vi "ListAttributes.vi"(6 "Inheritable Only? (F: all)":bool, 8 "error in (no error)":errorcluster, 11 "SMO in":refnum<class "SMO.lvclass">) -> (0 "error out":errorcluster, 2 "[Attributes]":refnum<class "Attribute.lvclass">[](array[class]), 3 "SMO out":refnum<class "SMO.lvclass">)   [LabVIEW 2021, in "smo.lvlib" / "SMO.lvclass"]
uses:
  SMO.lvclass
  Support/Attribute/Attribute.lvclass
  SMO.lvclass/SMO.ctl
  Support/Attribute/Attribute.lvclass/Attribute.ctl
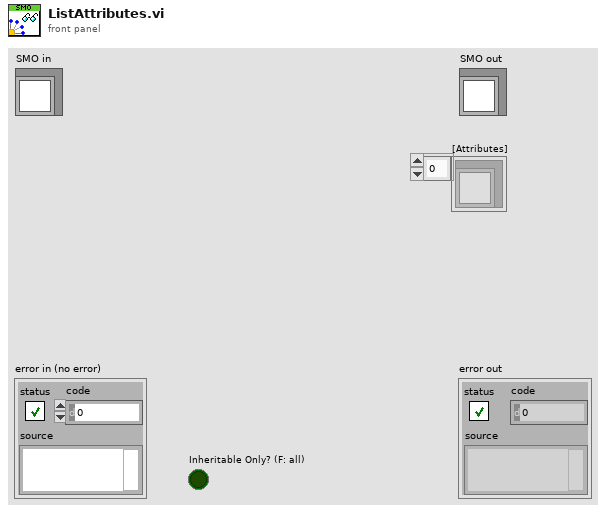
[diagram p1: front panel]
types:
  T1 = typedef "smo.lvlib/SMO.lvclass/PrivateData--Ref.ctl" = refnum<data-value>
  T2 = typedef "smo.lvlib/SMO.lvclass/PrivateData--Cluster.ctl" = cluster{"Parent Call":T3, "Registered Processes":T4[], "Sync Notifier":refnum<notifier>, "Process Error Notifier":refnum<notifier>, "Protected Events":T5, "Public Events":T6, "SMO State":T7, "[Attributes]":variant, "Launcher Close":refnum<notifier>, "Caller Watchdog":refnum<queue>, "Accessibility":T8, "NbStaticDependencies":u32}
  T3 = typedef "smo.lvlib/SMO.lvclass/Parent Call--Enum.ctl" = enum16{"Allows parent to run", "Does not request parent to run"}
  T4 = typedef "smo.lvlib/SMO.lvclass/RegisteredProcessData--Cluster.ctl" = cluster{"Name":string, "Static VI Ref":refnum<vi>, "Running":bool, "NotifierRef":u32}
  T5 = typedef "smo.lvlib/SMO.lvclass/Protected Events.ctl" = cluster{"StopProcesses":refnum<user-event>, "AbortProcesses":refnum<user-event>, "Config Changed":refnum<user-event>, "Dependency":refnum<user-event>}
  T6 = typedef "smo.lvlib/SMO.lvclass/Public Events.ctl" = cluster{"Error":refnum<user-event>, "State":refnum<user-event>, "Reserve State":refnum<user-event>}
  T7 = typedef "smo.lvlib/SMO.lvclass/SMOState --Enum.ctl" = enum16{"unknown", "Created", "Started", "Stopped"}
  T8 = typedef "smo.lvlib/SMO.lvclass/Accessibility--Cluster.ctl" = cluster{"Lock Key":string, "Reserve State":T9}
  T9 = typedef "smo.lvlib/SMO.lvclass/Reserve State--Enum.ctl" = enum16{"Unreserved", "Reserved", "Self-locked"}
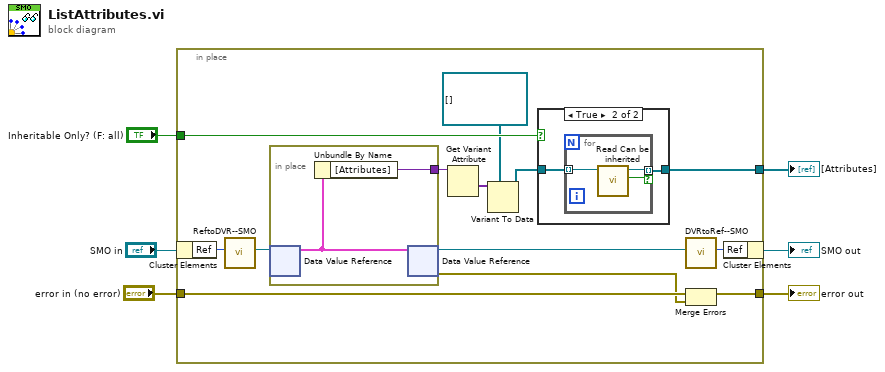
[diagram p0: block diagram]
diagram:
  n1 = in-place {
    in-place-border: "error in (no error)" -> [w15]
    in-place-border: [w13] -> w3
    in-place-border: [w11] -> w2
    in-place-border: "Inheritable Only? (F: all)" -> [w12]
    n2 = in-place-cluster #1("SMO in") -> ("Ref"=w19:u32)
    n3 = call "ReftoDVR--SMO.vi"("Ref"=w19) -> ("Ref"=w18:T1)  [unwired: 10 in]
    n4 = in-place {
      in-place-border: [w26] -> w10
      n5 = in-place-dvr #2(w18) -> (w27:T2)  [unwired: 1 out]
      n6 = Unbundle By Name(w27) -> ("[Attributes]"=w26:variant)
      n7 = in-place-dvr #2(w27) -> (w17:T1, w14:errorcluster)
    }
    n8 = Get Variant Attribute(Variant=w10) -> (values=w9:variant[])  [unwired: 3 in, 3 out]
    n9 = Variant To Data(type=refnum<class "Attribute.lvclass">[] [], Variant=w9) -> (data=w7:refnum<class "Attribute.lvclass">[])  [unwired: 1 in, 1 out]
    n10 = case shown="True" w12 {
      tunnel: w7 -> [w20 w22]
      tunnel: [w20 w21] -> w11
      frame False {
      }
      frame True {
        n11 = for {
          tunnel: w22 -> [w25] mode=indexing
          tunnel: [w24] -> w21 mode=indexing if=w23
          n12 = call "Read Can be inherited.vi"("Attribute in"=w25) -> ("Can be inherited"=w23:bool, "Attribute out"=w24:refnum<class "Attribute.lvclass">)  [unwired: 8 in, 1 out]
        }
      }
    }
    n13 = call "DVRtoRef--SMO.vi"("Ref"=w17) -> ("Ref"=w16:u32)  [unwired: 10 in]
    n14 = Merge Errors(w15, w14) -> (w13:errorcluster)
    n15 = in-place-cluster #1("Ref"=w16) -> (→"SMO out":refnum<class "SMO.lvclass">)
  }
  "error out" <- w3
  "[Attributes]" <- w2
